vi "FGV EventLog.vi"(2 "Action":enum16{"Reset", "Enqueue", "Dequeue"}(ring)=enum."Enqueue", 3 "String to log":string) -> (1 "Logging":string[](array[string]))   [LabVIEW 2020, in "WSsupport.lvlib"]
uses:
  WSsupport.lvlib
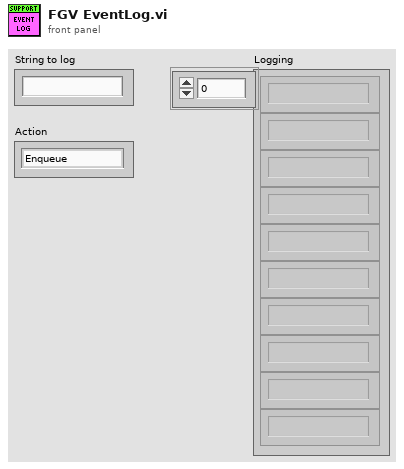
[diagram p1: front panel]
types:
  T1 = enum16{"open", "replace", "create", "open or create", "replace or create", "replace or create with confirmation"}
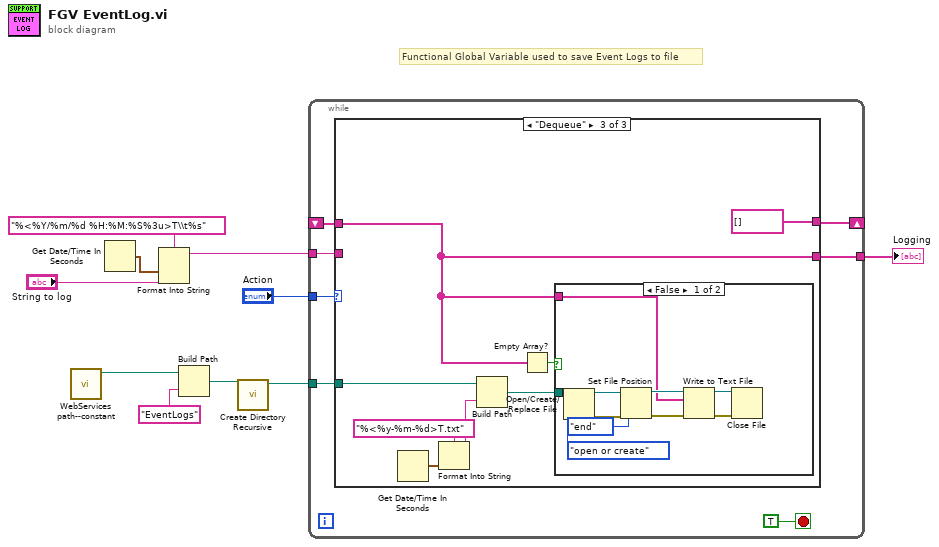
[diagram p0: block diagram]
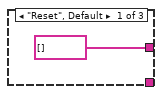
[diagram p2: hidden frame]
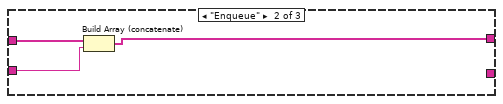
[diagram p3: hidden frame]
diagram:
  # "Functional Global Variable used to save Event Logs to file"
  n1 = call "WebServices path--constant.vi"() -> ("WebServices path"=w1:path)  [unwired: 11 in]
  n2 = Get Date/Time In Seconds() -> (seconds since 1Jan1904=w5:timestamp)
  n3 = Format Into String(format string="%<%Y/%m/%d %H:%M:%S%3u>T\\t%s", w5, "String to log") -> (resulting string=w2:string)  [unwired: 2 in, 1 out]
  n4 = Build Path(base path=w1, name or relative path="EventLogs") -> (appended path=w7:path)
  n5 = call <vilib>:"Create Directory Recursive.vi"("directory"=w7) -> ("directory copy"=w6:path)  [unwired: 4 in, 2 out]
  n6 = while {
    shift-right: [w15] -> _
    shift-left: _ -> [w14]
    tunnel: "Action" -> [w16]
    tunnel: w2 -> [w13]
    tunnel: [w12] -> w9
    tunnel: w6 -> [w11]
    stop <- TRUE stop-if-true
    n7 = case shown="\"Dequeue\"" w16 {
      tunnel: [string[] [] w19 string[] []] -> w15
      tunnel: w14 -> [_ w21 w23]
      tunnel: w13 -> [_ w20 _]
      tunnel: [_ _ w23] -> w12
      tunnel: w11 -> [_ _ w22]
      frame "Reset", Default {
      }
      frame "Enqueue" {
        n8 = Build Array (concatenate)(w21, w20) -> (w19:string[])
      }
      frame "Dequeue" {
        n9 = Get Date/Time In Seconds() -> (seconds since 1Jan1904=w28:timestamp)
        n10 = Format Into String(format string="%<%y-%m-%d>T.txt", w28) -> (resulting string=w26:string)  [unwired: 2 in, 1 out]
        n11 = Build Path(base path=w22, name or relative path=w26) -> (appended path=w25:path)
        n12 = Empty Array?(array=w23) -> (empty?=w24:bool)
        n13 = case shown="False" w24 {
          tunnel: w25 -> [w39 _]
          tunnel: w23 -> [w30 _]
          frame False {
            n14 = Open/Create/Replace File(file path (use dialog)=w39, operation (0:open)=T1."open or create") -> (refnum out=w37:refnum<file>, error out=w36:errorcluster)  [unwired: 4 in, 1 out]
            n15 = Set File Position(refnum=w37, from (0:start)=enum16{"start", "end", "current"}."end", error in=w36) -> (refnum out=w34:refnum<file>, error out=w33:errorcluster)  [unwired: 1 in]
            n16 = Write to Text File(file (use dialog)=w34, text=w30, error in=w33) -> (refnum out=w32:refnum<file>, error out=w31:errorcluster)  [unwired: 1 in, 1 out]
            n17 = Close File(refnum=w32, error in=w31) -> ()  [unwired: 2 out]
          }
          frame True {
          }
        }
      }
    }
  }
  "Logging" <- w9
